vi "Text Callback.vi"(4 "Front Panel Text Ref":refnum<vi>, 5 "Event Data":cluster{"sender":refnum<k24>, "e":refnum<k24>}, 6 "Control Ref":refnum<k24>, 7 "Event Common Data":T1) -> ()   [LabVIEW 2022 SP3]
uses:
  System.Speech
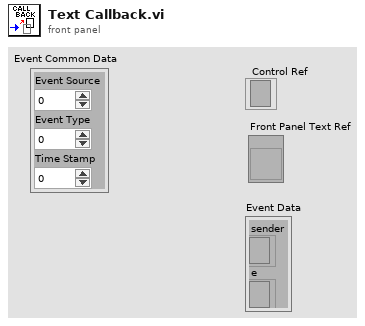
[diagram p1: front panel]
types:
  T1 = cluster{"Event Source":i32, "Event Type":u32, "Time Stamp":u32}
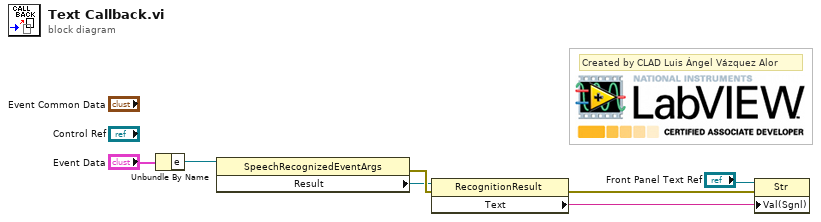
[diagram p0: block diagram]
diagram:
  # "Created by CLAD Luis Ángel Vázquez Alor"
  n1 = Unbundle By Name("Event Data") -> ("e"=w7:refnum<k24>)
  n2 = property class="SpeechRecognizedEventArgs"(reference=w7) -> (error out=w2:errorcluster, "Result"=w1:refnum<k24>)  [unwired: 1 in, 1 out]
  n3 = property class="RecognitionResult"(reference=w1, error in=w2) -> (error out=w6:errorcluster, "Text"=w5:string)  [unwired: 1 out]
  n4 = property class="Str"(reference="Front Panel Text Ref", error in=w6, "Val(Sgnl)"=w5) -> ()  [unwired: 2 out]
